vi "DSF.Engine.Timing.Set Decimation.vi"(10 "Decimation":u64=1, 11 "Timing in":refnum<class "DSF.Engine.Timing.lvclass">) -> (3 "Timing out":refnum<class "DSF.Engine.Timing.lvclass">)   [LabVIEW 2017, in "DSF.Engine.lvlib" / "DSF.Engine.Timing.lvclass"]
uses:
  Engine/Classes/Timing/DSF.Engine.Timing.lvclass
  Engine/Classes/Timing/DSF.Engine.Timing.lvclass/DSF.Engine.Timing.ctl
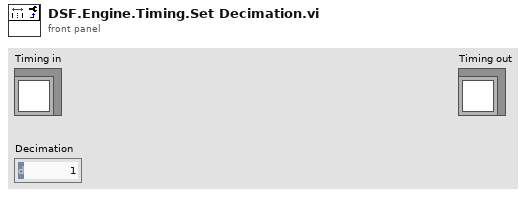
[diagram p1: front panel]
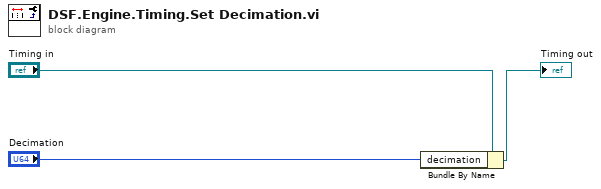
[diagram p0: block diagram]
diagram:
  n1 = Bundle By Name(cluster="Timing in", "decimation"="Decimation") -> (→"Timing out":refnum<class "DSF.Engine.Timing.lvclass">)
